vi "BUFMGR_bufs2str.vi"() -> (2 "buffers":string)   [LabVIEW 2016]
uses:
  BUFMGR_actionStruct.ctl
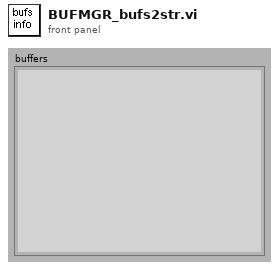
[diagram p1: front panel]
types:
  T1 = typedef "BUFMGR_actionStruct.ctl" = enum16{"get", "release", "get & lock", "unlock", "release all", "find", "release smaller than", "release bigger than", "release different than", "release equal to", "release unlocked", "info", "get & doublelock", "release secured", "double unlock"}
  T2 = typedef "BufferStruct.ctl" = cluster{"Name":string, "size (bytes)":u64, "pointer":u64, "Lock":bool, "slock":bool}
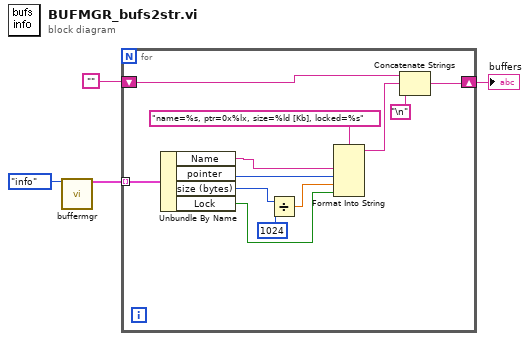
[diagram p0: block diagram]
diagram:
  n1 = call "buffermgr.vi"("Action"=BUFMGR_actionStruct."info") -> ("output buffers"=w3:T2[])  [unwired: 4 in, 10 out]
  n2 = for {
    tunnel: w3 -> [w16] mode=indexing
    shift-right: [w7] -> w1
    shift-left: "" -> [w6]
    n3 = Unbundle By Name(w16) -> ("Name"=w14:string, "pointer"=w13:u64, "size (bytes)"=w12:u64, "Lock"=w9:bool)
    n4 = Divide(x=w12, y=u64 1024) -> (x/y=w10:dbl)
    n5 = Format Into String(format string="name=%s, ptr=0x%lx, size=%ld [Kb], locked=%s", w14, w13, w10, w9) -> (resulting string=w8:string)  [unwired: 2 in, 1 out]
    n6 = Concatenate Strings(w6, w8, "\n") -> (w7:string)
  }
  "buffers" <- w1
